vi "Add to array if not in array.vi"(10 "Array in":u32[](array[numeric]), 11 "Number to add":u32) -> (2 "New array size":i32, 3 "Array out":u32[](array[numeric]))   [LabVIEW 2013]
panel:
  # "add client to list if not there already"
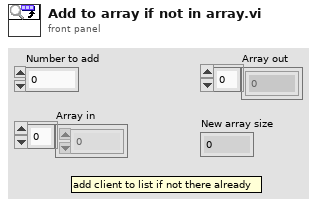
[diagram p1: front panel]
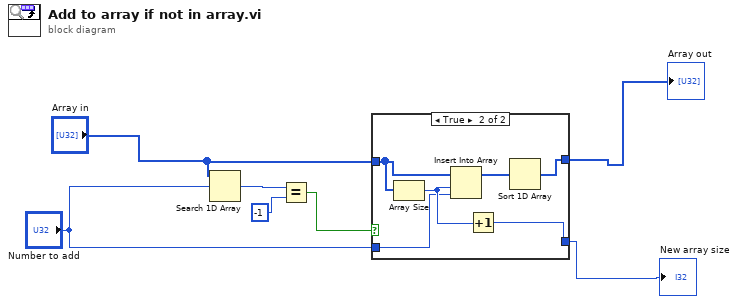
[diagram p0: block diagram]
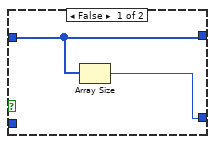
[diagram p2: hidden frame]
diagram:
  n1 = Search 1D Array(1D array="Array in", element="Number to add") -> (index of element=w1:i32)  [unwired: 1 in]
  n2 = Equal?(x=w1, y=-1) -> (x = y?=w3:bool)
  n3 = case shown="True" w3 {
    tunnel: "Array in" -> [w9 w15]
    tunnel: "Number to add" -> [_ w13]
    tunnel: [w8 w12] -> w6
    tunnel: [w9 w10] -> w7
    frame False {
      n4 = Array Size(array=w9) -> (size(s)=w8:i32)
    }
    frame True {
      n5 = Array Size(array=w15) -> (size(s)=w14:i32)
      n6 = Insert Into Array(array=w15, index=w14, new element=w13) -> (w11:u32[])
      n7 = Increment(x=w14) -> (x+1=w12:i32)
      n8 = Sort 1D Array(array=w11) -> (sorted array=w10:u32[])
    }
  }
  "Array out" <- w7
  "New array size" <- w6
